vi "Main.vi"() -> (0 "error out":errorcluster)   [LabVIEW 2019]
uses:
  <instrlib>/niDMM/nidmm.llb/niDMM Function.ctl
  <instrlib>/niSwitch/niSwitch.llb/niSwitch Topologies.ctl
  Utility/Result.ctl
  Utility/ErrorOutData.ctl
  <instrlib>/niDCPower/nidcpower.llb/niDCPower Send Software Edge Trigger - Signal.ctl
  <instrlib>/niDMM/nidmm.llb/niDMM Trigger.ctl
  <instrlib>/niDMM/nidmm.llb/niDMM Slope.ctl
  <instrlib>/niDMM/nidmm.llb/niDMM Sample Trigger.ctl
  <instrlib>/niDMM/nidmm.llb/niDMM Control Actions.ctl
  <instrlib>/niDCPower/nidcpower.llb/niDCPower Export Signal - Signal.ctl
  <instrlib>/niDMM/nidmm.llb/niDMM Configure Measurement Absolute.vi
  <instrlib>/niDCPower/nidcpower.llb/niDCPower Configure Software Edge Start Trigger.vi
  <instrlib>/niDCPower/nidcpower.llb/niDCPower Configure Software Edge Sequence Advance Trigger.vi
  <instrlib>/niSwitch/niSwitch.llb/niSwitch Connect Channels (Single).vi
  <instrlib>/niSwitch/niSwitch.llb/niSwitch Disconnect Channels (Single).vi
panel:
  in  "SMU Source Mode":i32(ring)=1021 items=["Single Point"=1020, "Sequence"=1021]
  in  "SMU Output Function":i32(ring)=1007 items=["DC Voltage"=1006, "DC Current"=1007, "Pulse Voltage"=1049, "Pulse Current"=1050]
  in  "SMU Sequence Name":string="MySequence"
  out "Channel Connected":string="ch63"
  in  "Default Results":T1[](array[typedef])
  out "All Results":T1[](array[typedef])=[{"Positive Voltage"=0.05015811388300842, "Positive Current"=0.0, "Negative Voltage"=0.05012649110640674, "Negative Current"=0.0, "Impedance"=inf, "ErrorOutData"={"Error Code"=-2, "Error Message"="\rDMM HI SENSE or LO SENSE lead disconnected\n- DMM measures NaN, or \n- DMM overrange warning, or\n- DMM voltage > DMM Voltage Fault Upper Limit "}}, {"Positive Voltage"=0.05018973665961011, "Positive Current"=0.0, "Negative Voltage"=0.05015811388300842, "Negative Current"=0.0, "Impedance"=inf, "ErrorOutData"={"Error Code"=-2, "Error Message"="\rDMM HI SENSE or LO SENSE lead disconnected\n- DMM measures NaN, or \n- DMM overrange warning, or\n- DMM voltage > DMM Voltage Fault Upper Limit "}}, {"Positive Voltage"=0.05009486832980505, "Positive Current"=0.0, "Negative Voltage"=0.05025298221281347, "Negative Current"=0.0, "Impedance"=-inf, "ErrorOutData"={"Error Code"=-2, "Error Message"="\rDMM HI SENSE or LO SENSE lead disconnected\n- DMM measures NaN, or \n- DMM overrange warning, or\n- DMM voltage > DMM Voltage Fault Upper Limit "}}, {"Positive Voltage"=0.05028460498941516, "Positive Current"=0.0, "Negative Voltage"=0.05, "Negative Current"=0.0, "Impedance"=inf, "ErrorOutData"={"Error Code"=-2, "Error Message"="\rDMM HI SENSE or LO SENSE lead disconnected\n- DMM measures NaN, or \n- DMM overrange warning, or\n- DMM voltage > DMM Voltage Fault Upper Limit "}}, {"Positive Voltage"=0.05025298221281347, "Positive Current"=0.0, "Negative Voltage"=0.05012649110640674, "Negative Current"=0.0, "Impedance"=inf, "ErrorOutData"={"Error Code"=-2, "Error Message"="\rDMM HI SENSE or LO SENSE lead disconnected\n- DMM measures NaN, or \n- DMM overrange warning, or\n- DMM voltage > DMM Voltage Fault Upper Limit "}}, {"Positive Voltage"=0.05015811388300842, "Positive Current"=0.0, "Negative Voltage"=0.05028460498941516, "Negative Current"=0.0, "Impedance"=-inf, "ErrorOutData"={"Error Code"=-2, "Error Message"="\rDMM HI SENSE or LO SENSE lead disconnected\n- DMM measures NaN, or \n- DMM overrange warning, or\n- DMM voltage > DMM Voltage Fault Upper Limit "}}, {"Positive Voltage"=0.05006324555320337, "Positive Current"=0.0, "Negative Voltage"=0.05015811388300842, "Negative Current"=0.0, "Impedance"=-inf, "ErrorOutData"={"Error Code"=-2, "Error Message"="\rDMM HI SENSE or LO SENSE lead disconnected\n- DMM measures NaN, or \n- DMM overrange warning, or\n- DMM voltage > DMM Voltage Fault Upper Limit "}}, {"Positive Voltage"=0.05006324555320337, "Positive Current"=0.0, "Negative Voltage"=0.05006324555320337, "Negative Current"=0.0, "Impedance"=nan, "ErrorOutData"={"Error Code"=-2, "Error Message"="\rDMM HI SENSE or LO SENSE lead disconnected\n- DMM measures NaN, or \n- DMM overrange warning, or\n- DMM voltage > DMM Voltage Fault Upper Limit "}}, {"Positive Voltage"=0.05018973665961011, "Positive Current"=0.0, "Negative Voltage"=0.05022135943621179, "Negative Current"=0.0, "Impedance"=-inf, "ErrorOutData"={"Error Code"=-2, "Error Message"="\rDMM HI SENSE or LO SENSE lead disconnected\n- DMM measures NaN, or \n- DMM overrange warning, or\n- DMM voltage > DMM Voltage Fault Upper Limit "}}, {"Positive Voltage"=0.05006324555320337, "Positive Current"=0.0, "Negative Voltage"=0.05025298221281347, "Negative Current"=0.0, "Impedance"=-inf, "ErrorOutData"={"Error Code"=-2, "Error Message"="\rDMM HI SENSE or LO SENSE lead disconnected\n- DMM measures NaN, or \n- DMM overrange warning, or\n- DMM voltage > DMM Voltage Fault Upper Limit "}}, {"Positive Voltage"=0.05018973665961011, "Positive Current"=0.0, "Negative Voltage"=0.05006324555320337, "Negative Current"=0.0, "Impedance"=inf, "ErrorOutData"={"Error Code"=-2, "Error Message"="\rDMM HI SENSE or LO SENSE lead disconnected\n- DMM measures NaN, or \n- DMM overrange warning, or\n- DMM voltage > DMM Voltage Fault Upper Limit "}}, {"Positive Voltage"=0.050031622776601684, "Positive Current"=0.0, "Negative Voltage"=0.05, "Negative Current"=0.0, "Impedance"=inf, "ErrorOutData"={"Error Code"=-2, "Error Message"="\rDMM HI SENSE or LO SENSE lead disconnected\n- DMM measures NaN, or \n- DMM overrange warning, or\n- DMM voltage > DMM Voltage Fault Upper Limit "}}, {"Positive Voltage"=0.05022135943621179, "Positive Current"=0.0, "Negative Voltage"=0.05015811388300842, "Negative Current"=0.0, "Impedance"=inf, "ErrorOutData"={"Error Code"=-2, "Error Message"="\rDMM HI SENSE or LO SENSE lead disconnected\n- DMM measures NaN, or \n- DMM overrange warning, or\n- DMM voltage > DMM Voltage Fault Upper Limit "}}, {"Positive Voltage"=0.05009486832980505, "Positive Current"=0.0, "Negative Voltage"=0.05009486832980505, "Negative Current"=0.0, "Impedance"=nan, "ErrorOutData"={"Error Code"=-2, "Error Message"="\rDMM HI SENSE or LO SENSE lead disconnected\n- DMM measures NaN, or \n- DMM overrange warning, or\n- DMM voltage > DMM Voltage Fault Upper Limit "}}, {"Positive Voltage"=0.05022135943621179, "Positive Current"=0.0, "Negative Voltage"=0.05025298221281347, "Negative Current"=0.0, "Impedance"=-inf, "ErrorOutData"={"Error Code"=-2, "Error Message"="\rDMM HI SENSE or LO SENSE lead disconnected\n- DMM measures NaN, or \n- DMM overrange warning, or\n- DMM voltage > DMM Voltage Fault Upper Limit "}}, {"Positive Voltage"=0.05028460498941516, "Positive Current"=0.0, "Negative Voltage"=0.05009486832980505, "Negative Current"=0.0, "Impedance"=inf, "ErrorOutData"={"Error Code"=-2, "Error Message"="\rDMM HI SENSE or LO SENSE lead disconnected\n- DMM measures NaN, or \n- DMM overrange warning, or\n- DMM voltage > DMM Voltage Fault Upper Limit "}}, {"Positive Voltage"=0.050031622776601684, "Positive Current"=0.0, "Negative Voltage"=0.05006324555320337, "Negative Current"=0.0, "Impedance"=-inf, "ErrorOutData"={"Error Code"=-2, "Error Message"="\rDMM HI SENSE or LO SENSE lead disconnected\n- DMM measures NaN, or \n- DMM overrange warning, or\n- DMM voltage > DMM Voltage Fault Upper Limit "}}, {"Positive Voltage"=0.05025298221281347, "Positive Current"=0.0, "Negative Voltage"=0.05025298221281347, "Negative Current"=0.0, "Impedance"=nan, "ErrorOutData"={"Error Code"=-2, "Error Message"="\rDMM HI SENSE or LO SENSE lead disconnected\n- DMM measures NaN, or \n- DMM overrange warning, or\n- DMM voltage > DMM Voltage Fault Upper Limit "}}, {"Positive Voltage"=0.05028460498941516, "Positive Current"=0.0, "Negative Voltage"=0.05015811388300842, "Negative Current"=0.0, "Impedance"=inf, "ErrorOutData"={"Error Code"=-2, "Error Message"="\rDMM HI SENSE or LO SENSE lead disconnected\n- DMM measures NaN, or \n- DMM overrange warning, or\n- DMM voltage > DMM Voltage Fault Upper Limit "}}, {"Positive Voltage"=0.05018973665961011, "Positive Current"=0.0, "Negative Voltage"=0.050031622776601684, "Negative Current"=0.0, "Impedance"=inf, "ErrorOutData"={"Error Code"=-2, "Error Message"="\rDMM HI SENSE or LO SENSE lead disconnected\n- DMM measures NaN, or \n- DMM overrange warning, or\n- DMM voltage > DMM Voltage Fault Upper Limit "}}, {"Positive Voltage"=0.05015811388300842, "Positive Current"=0.0, "Negative Voltage"=0.05, "Negative Current"=0.0, "Impedance"=inf, "ErrorOutData"={"Error Code"=-2, "Error Message"="\rDMM HI SENSE or LO SENSE lead disconnected\n- DMM measures NaN, or \n- DMM overrange warning, or\n- DMM voltage > DMM Voltage Fault Upper Limit "}}, {"Positive Voltage"=0.05018973665961011, "Positive Current"=0.0, "Negative Voltage"=0.05015811388300842, "Negative Current"=0.0, "Impedance"=inf, "ErrorOutData"={"Error Code"=-2, "Error Message"="\rDMM HI SENSE or LO SENSE lead disconnected\n- DMM measures NaN, or \n- DMM overrange warning, or\n- DMM voltage > DMM Voltage Fault Upper Limit "}}, {"Positive Voltage"=0.05018973665961011, "Positive Current"=0.0, "Negative Voltage"=0.05028460498941516, "Negative Current"=0.0, "Impedance"=-inf, "ErrorOutData"={"Error Code"=-2, "Error Message"="\rDMM HI SENSE or LO SENSE lead disconnected\n- DMM measures NaN, or \n- DMM overrange warning, or\n- DMM voltage > DMM Voltage Fault Upper Limit "}}, {"Positive Voltage"=0.05018973665961011, "Positive Current"=0.0, "Negative Voltage"=0.05028460498941516, "Negative Current"=0.0, "Impedance"=-inf, "ErrorOutData"={"Error Code"=-2, "Error Message"="\rDMM HI SENSE or LO SENSE lead disconnected\n- DMM measures NaN, or \n- DMM overrange warning, or\n- DMM voltage > DMM Voltage Fault Upper Limit "}}, {"Positive Voltage"=0.05028460498941516, "Positive Current"=0.0, "Negative Voltage"=0.05015811388300842, "Negative Current"=0.0, "Impedance"=inf, "ErrorOutData"={"Error Code"=-2, "Error Message"="\rDMM HI SENSE or LO SENSE lead disconnected\n- DMM measures NaN, or \n- DMM overrange warning, or\n- DMM voltage > DMM Voltage Fault Upper Limit "}}, {"Positive Voltage"=0.05, "Positive Current"=0.0, "Negative Voltage"=0.05022135943621179, "Negative Current"=0.0, "Impedance"=-inf, "ErrorOutData"={"Error Code"=-2, "Error Message"="\rDMM HI SENSE or LO SENSE lead disconnected\n- DMM measures NaN, or \n- DMM overrange warning, or\n- DMM voltage > DMM Voltage Fault Upper Limit "}}, {"Positive Voltage"=0.05, "Positive Current"=0.0, "Negative Voltage"=0.05018973665961011, "Negative Current"=0.0, "Impedance"=-inf, "ErrorOutData"={"Error Code"=-2, "Error Message"="\rDMM HI SENSE or LO SENSE lead disconnected\n- DMM measures NaN, or \n- DMM overrange warning, or\n- DMM voltage > DMM Voltage Fault Upper Limit "}}, {"Positive Voltage"=0.05022135943621179, "Positive Current"=0.0, "Negative Voltage"=0.05028460498941516, "Negative Current"=0.0, "Impedance"=-inf, "ErrorOutData"={"Error Code"=-2, "Error Message"="\rDMM HI SENSE or LO SENSE lead disconnected\n- DMM measures NaN, or \n- DMM overrange warning, or\n- DMM voltage > DMM Voltage Fault Upper Limit "}}, {"Positive Voltage"=0.05009486832980505, "Positive Current"=0.0, "Negative Voltage"=0.05, "Negative Current"=0.0, "Impedance"=inf, "ErrorOutData"={"Error Code"=-2, "Error Message"="\rDMM HI SENSE or LO SENSE lead disconnected\n- DMM measures NaN, or \n- DMM overrange warning, or\n- DMM voltage > DMM Voltage Fault Upper Limit "}}, {"Positive Voltage"=0.05012649110640674, "Positive Current"=0.0, "Negative Voltage"=0.05006324555320337, "Negative Current"=0.0, "Impedance"=inf, "ErrorOutData"={"Error Code"=-2, "Error Message"="\rDMM HI SENSE or LO SENSE lead disconnected\n- DMM measures NaN, or \n- DMM overrange warning, or\n- DMM voltage > DMM Voltage Fault Upper Limit "}}, {"Positive Voltage"=0.05, "Positive Current"=0.0, "Negative Voltage"=0.05, "Negative Current"=0.0, "Impedance"=nan, "ErrorOutData"={"Error Code"=-2, "Error Message"="\rDMM HI SENSE or LO SENSE lead disconnected\n- DMM measures NaN, or \n- DMM overrange warning, or\n- DMM voltage > DMM Voltage Fault Upper Limit "}}, {"Positive Voltage"=0.05, "Positive Current"=0.0, "Negative Voltage"=0.05012649110640674, "Negative Current"=0.0, "Impedance"=-inf, "ErrorOutData"={"Error Code"=-2, "Error Message"="\rDMM HI SENSE or LO SENSE lead disconnected\n- DMM measures NaN, or \n- DMM overrange warning, or\n- DMM voltage > DMM Voltage Fault Upper Limit "}}, {"Positive Voltage"=0.05015811388300842, "Positive Current"=0.0, "Negative Voltage"=0.05018973665961011, "Negative Current"=0.0, "Impedance"=-inf, "ErrorOutData"={"Error Code"=-2, "Error Message"="\rDMM HI SENSE or LO SENSE lead disconnected\n- DMM measures NaN, or \n- DMM overrange warning, or\n- DMM voltage > DMM Voltage Fault Upper Limit "}}, {"Positive Voltage"=0.05015811388300842, "Positive Current"=0.0, "Negative Voltage"=0.05018973665961011, "Negative Current"=0.0, "Impedance"=-inf, "ErrorOutData"={"Error Code"=-2, "Error Message"="\rDMM HI SENSE or LO SENSE lead disconnected\n- DMM measures NaN, or \n- DMM overrange warning, or\n- DMM voltage > DMM Voltage Fault Upper Limit "}}, {"Positive Voltage"=0.05022135943621179, "Positive Current"=0.0, "Negative Voltage"=0.05018973665961011, "Negative Current"=0.0, "Impedance"=inf, "ErrorOutData"={"Error Code"=-2, "Error Message"="\rDMM HI SENSE or LO SENSE lead disconnected\n- DMM measures NaN, or \n- DMM overrange warning, or\n- DMM voltage > DMM Voltage Fault Upper Limit "}}, {"Positive Voltage"=0.05, "Positive Current"=0.0, "Negative Voltage"=0.05018973665961011, "Negative Current"=0.0, "Impedance"=-inf, "ErrorOutData"={"Error Code"=-2, "Error Message"="\rDMM HI SENSE or LO SENSE lead disconnected\n- DMM measures NaN, or \n- DMM overrange warning, or\n- DMM voltage > DMM Voltage Fault Upper Limit "}}, {"Positive Voltage"=0.05028460498941516, "Positive Current"=0.0, "Negative Voltage"=0.05015811388300842, "Negative Current"=0.0, "Impedance"=inf, "ErrorOutData"={"Error Code"=-2, "Error Message"="\rDMM HI SENSE or LO SENSE lead disconnected\n- DMM measures NaN, or \n- DMM overrange warning, or\n- DMM voltage > DMM Voltage Fault Upper Limit "}}, {"Positive Voltage"=0.05009486832980505, "Positive Current"=0.0, "Negative Voltage"=0.05015811388300842, "Negative Current"=0.0, "Impedance"=-inf, "ErrorOutData"={"Error Code"=-2, "Error Message"="\rDMM HI SENSE or LO SENSE lead disconnected\n- DMM measures NaN, or \n- DMM overrange warning, or\n- DMM voltage > DMM Voltage Fault Upper Limit "}}, {"Positive Voltage"=0.05006324555320337, "Positive Current"=0.0, "Negative Voltage"=0.05, "Negative Current"=0.0, "Impedance"=inf, "ErrorOutData"={"Error Code"=-2, "Error Message"="\rDMM HI SENSE or LO SENSE lead disconnected\n- DMM measures NaN, or \n- DMM overrange warning, or\n- DMM voltage > DMM Voltage Fault Upper Limit "}}, {"Positive Voltage"=0.05018973665961011, "Positive Current"=0.0, "Negative Voltage"=0.05018973665961011, "Negative Current"=0.0, "Impedance"=nan, "ErrorOutData"={"Error Code"=-2, "Error Message"="\rDMM HI SENSE or LO SENSE lead disconnected\n- DMM measures NaN, or \n- DMM overrange warning, or\n- DMM voltage > DMM Voltage Fault Upper Limit "}}, {"Positive Voltage"=0.05012649110640674, "Positive Current"=0.0, "Negative Voltage"=0.050031622776601684, "Negative Current"=0.0, "Impedance"=inf, "ErrorOutData"={"Error Code"=-2, "Error Message"="\rDMM HI SENSE or LO SENSE lead disconnected\n- DMM measures NaN, or \n- DMM overrange warning, or\n- DMM voltage > DMM Voltage Fault Upper Limit "}}, {"Positive Voltage"=0.05012649110640674, "Positive Current"=0.0, "Negative Voltage"=0.05, "Negative Current"=0.0, "Impedance"=inf, "ErrorOutData"={"Error Code"=-2, "Error Message"="\rDMM HI SENSE or LO SENSE lead disconnected\n- DMM measures NaN, or \n- DMM overrange warning, or\n- DMM voltage > DMM Voltage Fault Upper Limit "}}, {"Positive Voltage"=0.050031622776601684, "Positive Current"=0.0, "Negative Voltage"=0.05015811388300842, "Negative Current"=0.0, "Impedance"=-inf, "ErrorOutData"={"Error Code"=-2, "Error Message"="\rDMM HI SENSE or LO SENSE lead disconnected\n- DMM measures NaN, or \n- DMM overrange warning, or\n- DMM voltage > DMM Voltage Fault Upper Limit "}}, {"Positive Voltage"=0.05012649110640674, "Positive Current"=0.0, "Negative Voltage"=0.05025298221281347, "Negative Current"=0.0, "Impedance"=-inf, "ErrorOutData"={"Error Code"=-2, "Error Message"="\rDMM HI SENSE or LO SENSE lead disconnected\n- DMM measures NaN, or \n- DMM overrange warning, or\n- DMM voltage > DMM Voltage Fault Upper Limit "}}, {"Positive Voltage"=0.05009486832980505, "Positive Current"=0.0, "Negative Voltage"=0.05028460498941516, "Negative Current"=0.0, "Impedance"=-inf, "ErrorOutData"={"Error Code"=-2, "Error Message"="\rDMM HI SENSE or LO SENSE lead disconnected\n- DMM measures NaN, or \n- DMM overrange warning, or\n- DMM voltage > DMM Voltage Fault Upper Limit "}}, {"Positive Voltage"=0.050031622776601684, "Positive Current"=0.0, "Negative Voltage"=0.05015811388300842, "Negative Current"=0.0, "Impedance"=-inf, "ErrorOutData"={"Error Code"=-2, "Error Message"="\rDMM HI SENSE or LO SENSE lead disconnected\n- DMM measures NaN, or \n- DMM overrange warning, or\n- DMM voltage > DMM Voltage Fault Upper Limit "}}, {"Positive Voltage"=0.05012649110640674, "Positive Current"=0.0, "Negative Voltage"=0.05, "Negative Current"=0.0, "Impedance"=inf, "ErrorOutData"={"Error Code"=-2, "Error Message"="\rDMM HI SENSE or LO SENSE lead disconnected\n- DMM measures NaN, or \n- DMM overrange warning, or\n- DMM voltage > DMM Voltage Fault Upper Limit "}}, {"Positive Voltage"=0.05012649110640674, "Positive Current"=0.0, "Negative Voltage"=0.05022135943621179, "Negative Current"=0.0, "Impedance"=-inf, "ErrorOutData"={"Error Code"=-2, "Error Message"="\rDMM HI SENSE or LO SENSE lead disconnected\n- DMM measures NaN, or \n- DMM overrange warning, or\n- DMM voltage > DMM Voltage Fault Upper Limit "}}, {"Positive Voltage"=0.05025298221281347, "Positive Current"=0.0, "Negative Voltage"=0.05015811388300842, "Negative Current"=0.0, "Impedance"=inf, "ErrorOutData"={"Error Code"=-2, "Error Message"="\rDMM HI SENSE or LO SENSE lead disconnected\n- DMM measures NaN, or \n- DMM overrange warning, or\n- DMM voltage > DMM Voltage Fault Upper Limit "}}, {"Positive Voltage"=0.05028460498941516, "Positive Current"=0.0, "Negative Voltage"=0.05006324555320337, "Negative Current"=0.0, "Impedance"=inf, "ErrorOutData"={"Error Code"=-2, "Error Message"="\rDMM HI SENSE or LO SENSE lead disconnected\n- DMM measures NaN, or \n- DMM overrange warning, or\n- DMM voltage > DMM Voltage Fault Upper Limit "}}, {"Positive Voltage"=0.050031622776601684, "Positive Current"=0.0, "Negative Voltage"=0.05025298221281347, "Negative Current"=0.0, "Impedance"=-inf, "ErrorOutData"={"Error Code"=-2, "Error Message"="\rDMM HI SENSE or LO SENSE lead disconnected\n- DMM measures NaN, or \n- DMM overrange warning, or\n- DMM voltage > DMM Voltage Fault Upper Limit "}}, {"Positive Voltage"=0.05015811388300842, "Positive Current"=0.0, "Negative Voltage"=0.05, "Negative Current"=0.0, "Impedance"=inf, "ErrorOutData"={"Error Code"=-2, "Error Message"="\rDMM HI SENSE or LO SENSE lead disconnected\n- DMM measures NaN, or \n- DMM overrange warning, or\n- DMM voltage > DMM Voltage Fault Upper Limit "}}, {"Positive Voltage"=0.05006324555320337, "Positive Current"=0.0, "Negative Voltage"=0.05009486832980505, "Negative Current"=0.0, "Impedance"=-inf, "ErrorOutData"={"Error Code"=-2, "Error Message"="\rDMM HI SENSE or LO SENSE lead disconnected\n- DMM measures NaN, or \n- DMM overrange warning, or\n- DMM voltage > DMM Voltage Fault Upper Limit "}}, {"Positive Voltage"=0.05012649110640674, "Positive Current"=0.0, "Negative Voltage"=0.05022135943621179, "Negative Current"=0.0, "Impedance"=-inf, "ErrorOutData"={"Error Code"=-2, "Error Message"="\rDMM HI SENSE or LO SENSE lead disconnected\n- DMM measures NaN, or \n- DMM overrange warning, or\n- DMM voltage > DMM Voltage Fault Upper Limit "}}, {"Positive Voltage"=0.05006324555320337, "Positive Current"=0.0, "Negative Voltage"=0.05, "Negative Current"=0.0, "Impedance"=inf, "ErrorOutData"={"Error Code"=-2, "Error Message"="\rDMM HI SENSE or LO SENSE lead disconnected\n- DMM measures NaN, or \n- DMM overrange warning, or\n- DMM voltage > DMM Voltage Fault Upper Limit "}}, {"Positive Voltage"=0.05, "Positive Current"=0.0, "Negative Voltage"=0.05, "Negative Current"=0.0, "Impedance"=nan, "ErrorOutData"={"Error Code"=-2, "Error Message"="\rDMM HI SENSE or LO SENSE lead disconnected\n- DMM measures NaN, or \n- DMM overrange warning, or\n- DMM voltage > DMM Voltage Fault Upper Limit "}}, {"Positive Voltage"=0.05028460498941516, "Positive Current"=0.0, "Negative Voltage"=0.05018973665961011, "Negative Current"=0.0, "Impedance"=inf, "ErrorOutData"={"Error Code"=-2, "Error Message"="\rDMM HI SENSE or LO SENSE lead disconnected\n- DMM measures NaN, or \n- DMM overrange warning, or\n- DMM voltage > DMM Voltage Fault Upper Limit "}}, {"Positive Voltage"=0.050031622776601684, "Positive Current"=0.0, "Negative Voltage"=0.05018973665961011, "Negative Current"=0.0, "Impedance"=-inf, "ErrorOutData"={"Error Code"=-2, "Error Message"="\rDMM HI SENSE or LO SENSE lead disconnected\n- DMM measures NaN, or \n- DMM overrange warning, or\n- DMM voltage > DMM Voltage Fault Upper Limit "}}, {"Positive Voltage"=0.05006324555320337, "Positive Current"=0.0, "Negative Voltage"=0.05006324555320337, "Negative Current"=0.0, "Impedance"=nan, "ErrorOutData"={"Error Code"=-2, "Error Message"="\rDMM HI SENSE or LO SENSE lead disconnected\n- DMM measures NaN, or \n- DMM overrange warning, or\n- DMM voltage > DMM Voltage Fault Upper Limit "}}, {"Positive Voltage"=0.05025298221281347, "Positive Current"=0.0, "Negative Voltage"=0.05015811388300842, "Negative Current"=0.0, "Impedance"=inf, "ErrorOutData"={"Error Code"=-2, "Error Message"="\rDMM HI SENSE or LO SENSE lead disconnected\n- DMM measures NaN, or \n- DMM overrange warning, or\n- DMM voltage > DMM Voltage Fault Upper Limit "}}, {"Positive Voltage"=0.05, "Positive Current"=0.0, "Negative Voltage"=0.05022135943621179, "Negative Current"=0.0, "Impedance"=-inf, "ErrorOutData"={"Error Code"=-2, "Error Message"="\rDMM HI SENSE or LO SENSE lead disconnected\n- DMM measures NaN, or \n- DMM overrange warning, or\n- DMM voltage > DMM Voltage Fault Upper Limit "}}, {"Positive Voltage"=0.05018973665961011, "Positive Current"=0.0, "Negative Voltage"=0.05, "Negative Current"=0.0, "Impedance"=inf, "ErrorOutData"={"Error Code"=-2, "Error Message"="\rDMM HI SENSE or LO SENSE lead disconnected\n- DMM measures NaN, or \n- DMM overrange warning, or\n- DMM voltage > DMM Voltage Fault Upper Limit "}}, {"Positive Voltage"=0.05018973665961011, "Positive Current"=0.0, "Negative Voltage"=0.05018973665961011, "Negative Current"=0.0, "Impedance"=nan, "ErrorOutData"={"Error Code"=-2, "Error Message"="\rDMM HI SENSE or LO SENSE lead disconnected\n- DMM measures NaN, or \n- DMM overrange warning, or\n- DMM voltage > DMM Voltage Fault Upper Limit "}}, {"Positive Voltage"=0.05022135943621179, "Positive Current"=0.0, "Negative Voltage"=0.05015811388300842, "Negative Current"=0.0, "Impedance"=inf, "ErrorOutData"={"Error Code"=-2, "Error Message"="\rDMM HI SENSE or LO SENSE lead disconnected\n- DMM measures NaN, or \n- DMM overrange warning, or\n- DMM voltage > DMM Voltage Fault Upper Limit "}}]
  out "Result":T1={"Positive Voltage"=0.05022135943621179, "Positive Current"=0.0, "Negative Voltage"=0.05015811388300842, "Negative Current"=0.0, "Impedance"=inf, "ErrorOutData"={"Error Code"=-2, "Error Message"="\rDMM HI SENSE or LO SENSE lead disconnected\n- DMM measures NaN, or \n- DMM overrange warning, or\n- DMM voltage > DMM Voltage Fault Upper Limit "}}
  out "Switch Channel List":string[](array[string])=["ch0", "ch1", "ch2", "ch3", "ch4", "ch5", "ch6", "ch7", "ch8", "ch9", "ch10", "ch11", "ch12", "ch13", "ch14", "ch15", "ch16", "ch17", "ch18", "ch19", "ch20", "ch21", "ch22", "ch23", "ch24", "ch25", "ch26", "ch27", "ch28", "ch29", "ch30", "ch31", "ch32", "ch33", "ch34", "ch35", "ch36", "ch37", "ch38", "ch39", "ch40", "ch41", "ch42", "ch43", "ch44", "ch45", "ch46", "ch47", "ch48", "ch49", "ch50", "ch51", "ch52", "ch53", "ch54", "ch55", "ch56", "ch57", "ch58", "ch59", "ch60", "ch61", "ch62", "ch63"]
  in  "SMU Sequence Number of Steps":i32=3
  in  "Sense MUX Switch Topology":T3="2530/2-Wire 64x1 Mux" caption="Sense MUX Topology"
  in  "Sense MUX Switch Resource Name":refnum<k15>="2530B"
  in  "Source MUX Switch Topology":T3="2575/2-Wire 98x1 Mux" caption="Source MUX Topology"
  in  "Source MUX Switch Resource Name":refnum<k15>="2575"
  in  "SMU Sequence Loop Count (Number of Welds)":i32=64
  in  "SMU Source Delay (s)":dbl=0.001 format="%#_13g"
  in  "SMU Measurement Aperture Time (s)":dbl=0.04 format="%#_13g"
  in  "SMU Voltage Limit Range (V)":dbl=6.0 format="%#_13g"
  in  "SMU Voltage Limit (V)":dbl=6.0 format="%#_13g"
  in  "SMU Current Level Range (A)":dbl=1.0 format="%#_13g"
  in  "SMU Current Level (A)":dbl=1.0 format="%#_13g"
  in  "SMU Advanced Sequence Properties":i32[](array[ring])=[1150009, 1150058, 1150051] caption="SMU Advanced Sequence - Step Properties" items=["Source -> Output Function"=1150008, "Source -> Output Enabled"=1250006, "Source -> Output Resistance"=1150061, "Source -> Transient Response"=1150062, "Source -> Custom Transient Response -> Voltage Gain Bandwidth"=1150067, "Source -> Custom Transient Response -> Voltage Compensation Frequency"=1150068, "Source -> Custom Transient Response -> Voltage Pole-Zero Ratio"=1150069, "Source -> Custom Transient Response -> Current Gain Bandwidth"=1150070, "Source -> Custom Transient Response -> Current Compensation Frequency"=1150071, "Source -> Custom Transient Response -> Current Pole-Zero Ratio"=1150072, "Source -> DC Voltage -> Voltage Level"=1250001, "Source -> DC Voltage -> Voltage Level Range"=1150005, "Source -> DC Voltage -> Current Limit"=1250005, "Source -> DC Voltage -> Current Limit High"=1150187, "Source -> DC Voltage -> Current Limit Low"=1150188, "Source -> DC Voltage -> Current Limit Range"=1150004, "Source -> DC Current -> Current Level"=1150009, "Source -> DC Current -> Current Level Range"=1150011, "Source -> DC Current -> Voltage Limit"=1150010, "Source -> DC Current -> Voltage Limit High"=1150185, "Source -> DC Current -> Voltage Limit Low"=1150186, "Source -> DC Current -> Voltage Limit Range"=1150012, "Source -> Pulse Voltage -> Pulse Voltage Level"=1150080, "Source -> Pulse Voltage -> Pulse Bias Voltage Level"=1150082, "Source -> Pulse Voltage -> Pulse Voltage Level Range"=1150084, "Source -> Pulse Voltage -> Pulse Current Limit"=1150081, "Source -> Pulse Voltage -> Pulse Current Limit High"=1150193, "Source -> Pulse Voltage -> Pulse Current Limit Low"=1150194, "Source -> Pulse Voltage -> Pulse Bias Current Limit"=1150083, "Source -> Pulse Voltage -> Pulse Bias Current Limit High"=1150195, "Source -> Pulse Voltage -> Pulse Bias Current Limit Low"=1150196, "Source -> Pulse Voltage -> Pulse Current Limit Range"=1150085, "Source -> Pulse Current -> Pulse Current Level"=1150086, "Source -> Pulse Current -> Pulse Bias Current Level"=1150088, "Source -> Pulse Current -> Pulse Current Level Range"=1150090, "Source -> Pulse Current -> Pulse Voltage Limit"=1150087, "Source -> Pulse Current -> Pulse Voltage Limit High"=1150189, "Source -> Pulse Current -> Pulse Voltage Limit Low"=1150190, "Source -> Pulse Current -> Pulse Bias Voltage Limit"=1150089, "Source -> Pulse Current -> Pulse Bias Voltage Limit High"=1150191, "Source -> Pulse Current -> Pulse Bias Voltage Limit Low"=1150192, "Source -> Pulse Current -> Pulse Voltage Limit Range"=1150091, "Source -> Advanced -> Source Delay"=1150051, "Source -> Advanced -> Pulse Bias Delay"=1150092, "Source -> Advanced -> Pulse On Time"=1150093, "Source -> Advanced -> Pulse Off Time"=1150094, "Source -> Advanced -> OVP Enabled"=1250002, "Source -> Advanced -> OVP Limit"=1250003, "Source -> Advanced -> Compliance Limit Symmetry"=1150184, "Source -> Advanced -> Sequence Step Delta Time"=1150198, "Measurement -> Sense"=1150013, "Measurement -> Aperture Time"=1150058, "Measurement -> Measure Record Length"=1150063, "Measurement -> Advanced -> DC Noise Rejection"=1150066, "Measurement -> Autorange"=1150244, "Measurement -> Advanced -> Autorange Behavior"=1150245, "Measurement -> Advanced -> Autorange Aperture Time Mode"=1150246, "Measurement -> Advanced -> Autorange Minimum Aperture Time"=1150247, "Measurement -> Advanced -> Autorange Minimum Aperture Time Units"=1105248]
  in  "DMM Range (V)":dbl=0.1 format="%#_13g"
  in  "DMM Function":T4
  in  "DMM Resource Name":refnum<k15>="DMM"
  in  "SMU Resource Name":refnum<k15>="SMU"
  in  "DMM Settle Time (s)":dbl=0.002 format="%#_13g"
  in  "DMM Aperture Time (s)":dbl=0.033 format="%#_13g"
  in  "Stop":bool
  out "Channel Index":i32=63
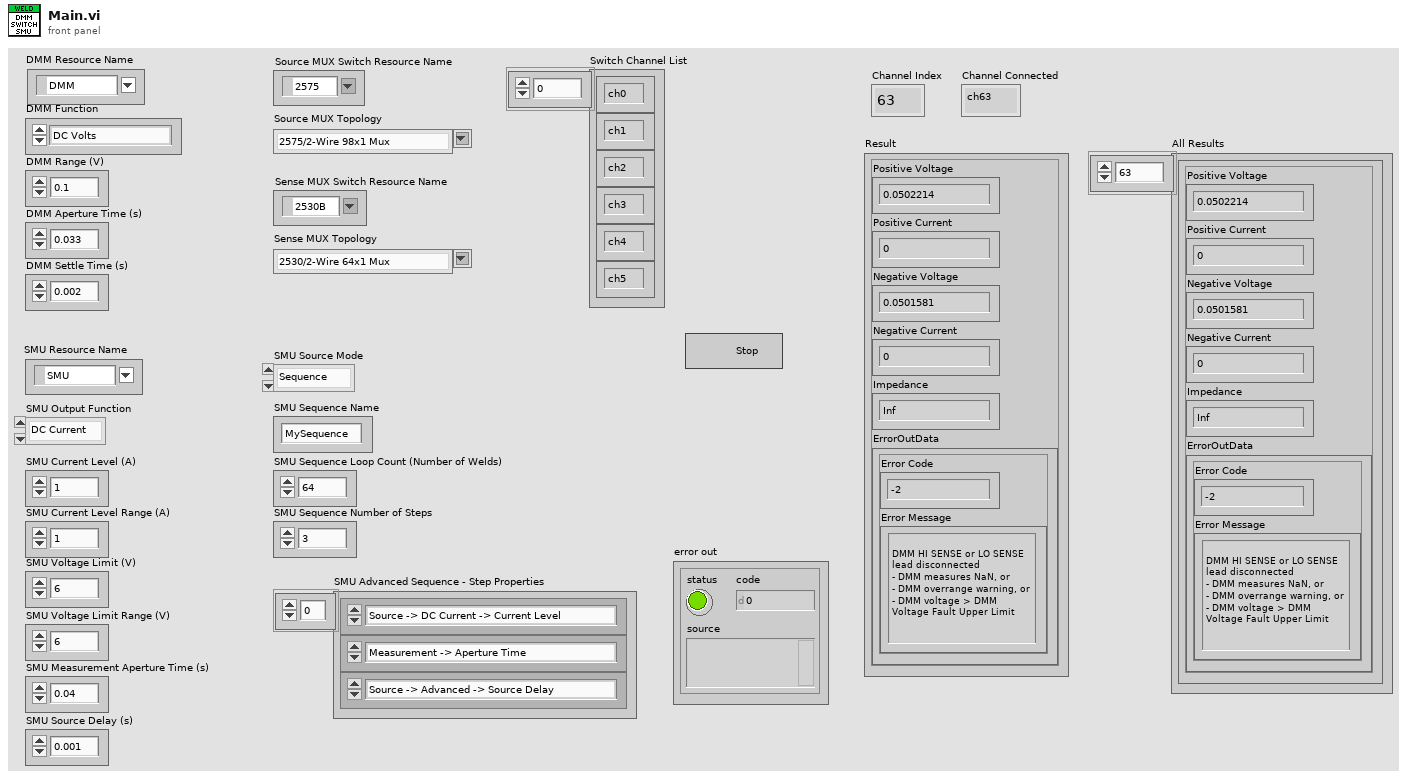
[diagram p1: front panel]
types:
  T1 = typedef "Result.ctl" = cluster{"Positive Voltage":dbl, "Positive Current":dbl, "Negative Voltage":dbl, "Negative Current":dbl, "Impedance":dbl, "ErrorOutData":T2}
  T2 = typedef "ErrorOutData.ctl" = cluster{"Error Code":i32, "Error Message":string}
  T3 = typedef "niSwitch Topologies.ctl" = string
  T4 = typedef "niDMM Function.ctl" = enum16{"DC Volts", "AC Volts", "DC Current", "AC Current", "2-wire Resistance", "4-wire Resistance", "Diode", "Frequency", "Period", "AC Volts DC Coupled", "Capacitance", "Inductance", "Temperature"}
  T5 = typedef "niDCPower Export Signal - Signal.ctl" = i32
  T6 = typedef "niDMM Control Actions.ctl" = i32
  T7 = typedef "niDMM Slope.ctl" = enum16{"Rising Edge", "Falling Edge"}
  T8 = typedef "niDMM Sample Trigger.ctl" = enum16{"Immediate", "External", "TTL 0", "TTL 1", "TTL 2", "TTL 3", "TTL 4", "TTL 5", "TTL 6", "Interval", "Software", "TTL 7", "PXI Star", "LBR Trig 1", "Aux Trig 1"}
  T9 = typedef "niDMM Trigger.ctl" = enum16{"Immediate", "External", "TTL 0", "TTL 1", "TTL 2", "TTL 3", "TTL 4", "TTL 5", "TTL 6", "Software", "TTL 7", "PXI Star", "LBR Trig 1", "Aux Trig 1"}
  T10 = typedef "niDCPower Send Software Edge Trigger - Signal.ctl" = i32
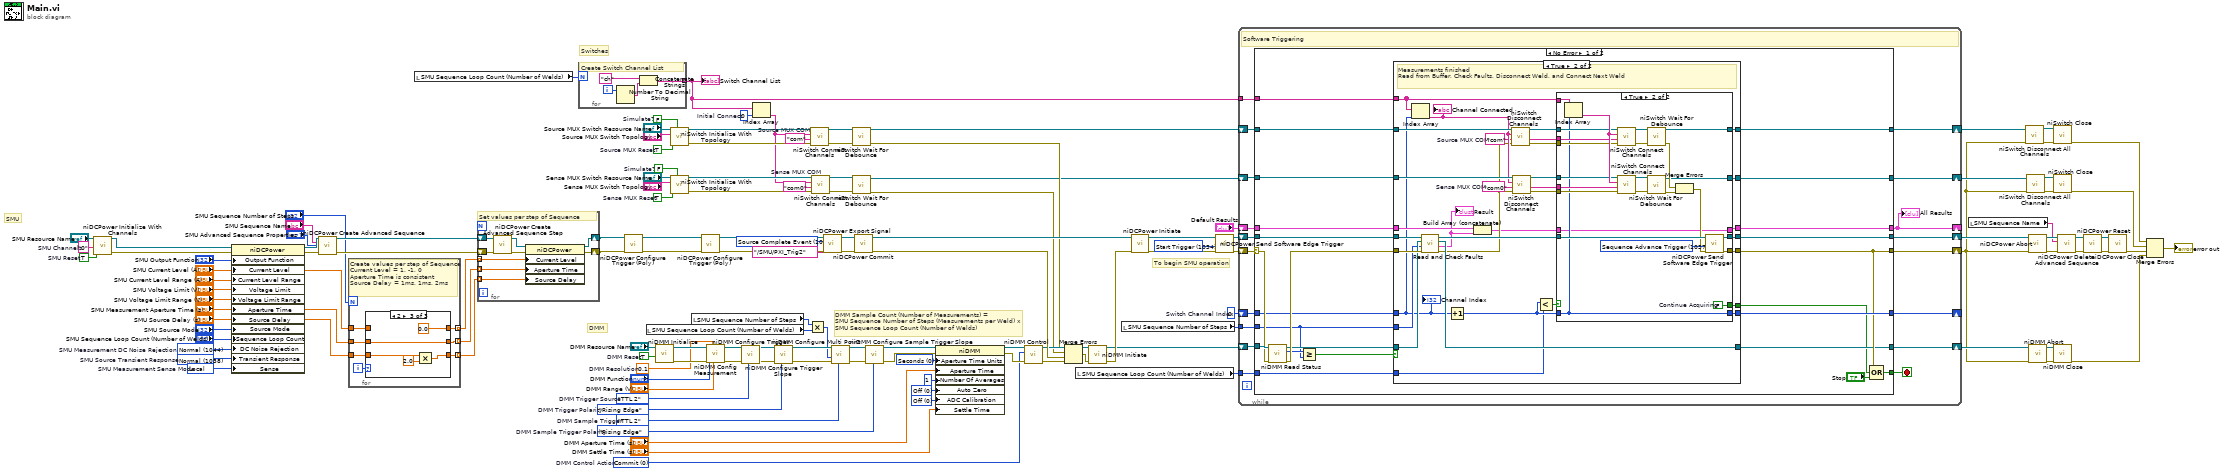
[diagram p0: block diagram]
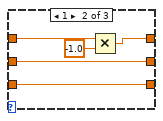
[diagram p3: hidden frame]
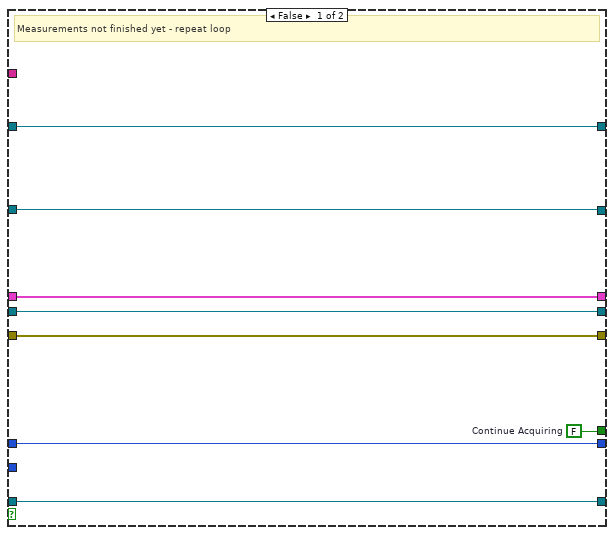
[diagram p4: hidden frame]
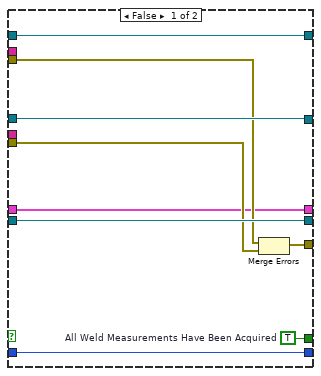
[diagram p5: hidden frame]
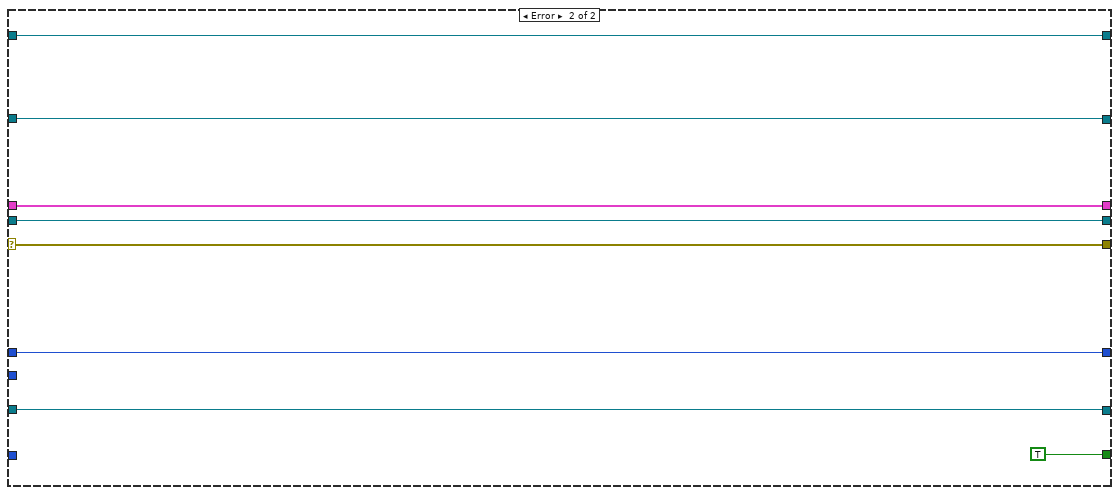
[diagram p6: hidden frame]
diagram:
  w29 = "com0"  # Sense MUX COM
  w30 = 0  # Initial Connect
  w31 = "com"  # Source MUX COM
  w36 = TRUE  # Sense MUX Reset
  w39 = FALSE  # Simulate?
  w40 = TRUE  # Source MUX Reset
  w43 = FALSE  # Simulate?
  w49 = T5 1030 items=["Source Complete Event"=1030, "Measure Complete Event"=1031, "Sequence Iteration Complete Event"=1032, "Sequence Engine Done Event"=1033, "Pulse Complete Event"=1051, "Ready For Pulse Trigger Event"=1052, "Start Trigger"=1034, "Source Trigger"=1035, "Measure Trigger"=1036, "Sequence Advance Trigger"=1037, "Pulse Trigger"=1053] ("signal")
  w65 = 1044 items=["Normal"=1044, "Second-Order"=1043]  # SMU Measurement DC Noise Rejection
  w61 = 1008 items=["Local"=1008, "Remote"=1009]  # SMU Measurement Sense Mode
  w62 = 1038 items=["Slow"=1041, "Normal"=1038, "Fast"=1039, "Custom"=1042]  # SMU Source Transient Response
  w75 = TRUE  # SMU Reset
  w76 = "0"  # SMU Channels
  w79 = 0 items=["Auto"=-1, "Off"=0, "On"=1] ("Configuration:Measurement Options:ADC Calibration")
  w80 = 0 items=["Auto"=-1, "Off"=0, "On"=1, "Once"=2] ("Configuration:Measurement Options:Auto Zero")
  w83 = 0 items=["Seconds", "Power Line Cycles"] ("Configuration:Advanced:Aperture Time Units")
  w84 = T6 0 items=["Commit"]  # DMM Control Action
  w93 = niDMM_Slope."Rising Edge"  # DMM Sample Trigger Polarity
  w97 = niDMM_Sample_Trigger."TTL 2"  # DMM Sample Trigger
  w100 = niDMM_Slope."Rising Edge"  # DMM Trigger Polarity
  w103 = niDMM_Trigger."TTL 2"  # DMM Trigger Source
  w106 = 0.1  # DMM Resolution
  w109 = TRUE  # DMM Reset
  w118 = 0  # Switch Channel Index
  w119 = T10 1034 items=["Start Trigger"=1034, "Source Trigger"=1035, "Measure Trigger"=1036, "Sequence Advance Trigger"=1037, "Pulse Trigger"=1053] ("signal")
  # "DMM Sample Count (Number of Measurements) = \nSMU Sequence Number of Steps (Measurements per Weld) x \nSMU Sequence Loop Count (Number of Welds)"
  # "DMM"
  # "SMU"
  # "Switches"
  # "To begin SMU operation"
  n1 = call <instrlib>:"niDCPower Initialize With Channels.vi"("reset (false)"=w75, "channels"=w76, "resource name"="SMU Resource Name") -> ("error out"=w63:errorcluster, "instrument handle out"=w64:refnum<k15>)  [unwired: 7 in]
  n2 = property class="niDCPower"(reference=w64, error in=w63, "Output Function"="SMU Output Function", "Current Level"="SMU Current Level (A)", "Current Level Range"="SMU Current Level Range (A)", "Voltage Limit"="SMU Voltage Limit (V)", "Voltage Limit Range"="SMU Voltage Limit Range (V)", "Aperture Time"="SMU Measurement Aperture Time (s)", "Source Delay"="SMU Source Delay (s)", "Source Mode"="SMU Source Mode", "Sequence Loop Count"="SMU Sequence Loop Count (Number of Welds)", "DC Noise Rejection"=w65, "Transient Response"=w62, "Sense"=w61) -> (reference out=w72:refnum<k15>, error out=w73:errorcluster)
  n3 = call <instrlib>:"niDCPower Create Advanced Sequence.vi"("instrument handle"=w72, "sequence name"="SMU Sequence Name", "advanced sequence properties"="SMU Advanced Sequence Properties", "error in (no error)"=w73) -> ("instrument handle out"=w60:refnum<k15>, "error out"=w59:errorcluster)  [unwired: 10 in]
  n4 = for {
    N: "SMU Sequence Number of Steps" -> [_]
    tunnel: "SMU Current Level (A)" -> [w141]
    tunnel: [w140] -> w56 mode=indexing
    tunnel: "SMU Measurement Aperture Time (s)" -> [w139]
    tunnel: [w138] -> w44 mode=indexing
    tunnel: "SMU Source Delay (s)" -> [w137]
    tunnel: [w136] -> w53 mode=indexing
    i -> [w142]
    # "Create values per step of Sequence\nCurrent Level = 1, -1, 0\nAperture Time is consistent\nSource Delay = 1ms, 1ms, 2ms"
    n5 = case shown="2" w142 {
      tunnel: w141 -> [w145 w149 _]
      tunnel: [w145 w150 0.0 ("current")] -> w140
      tunnel: w139 -> [w144 w147 w154]
      tunnel: [w144 w147 w154] -> w138
      tunnel: w137 -> [w143 w146 w152]
      tunnel: [w143 w146 w151] -> w136
      frame 0, Default {
      }
      frame 1 {
        n6 = Multiply(x=w149, y=-1.0) -> (x*y=w150:dbl)
      }
      frame 2 {
        n7 = Multiply(x=w152, y=2.0) -> (x*y=w151:dbl)
      }
    }
  }
  n8 = local read "SMU Sequence Loop Count (Number of Welds)"() -> (w34:i32)
  n9 = for {
    shift-right: [w161] -> w51
    shift-left: w59 -> [w164]
    shift-right: [w160] -> w52
    shift-left: w60 -> [w159]
    tunnel: w53 -> [w158] mode=indexing
    tunnel: w56 -> [w156] mode=indexing
    tunnel: w44 -> [w157] mode=indexing
    # "Set values per step of Sequence"
    n10 = call <instrlib>:"niDCPower Create Advanced Sequence Step.vi"("error in (no error)"=w164, "instrument handle"=w159) -> ("error out"=w162:errorcluster, "instrument handle out"=w163:refnum<k15>)  [unwired: 8 in]
    n11 = property class="niDCPower"(reference=w163, error in=w162, "Current Level"=w156, "Aperture Time"=w157, "Source Delay"=w158) -> (reference out=w160:refnum<k15>, error out=w161:errorcluster)
  }
  n12 = for {
    N: w34 -> [_]
    tunnel: [w165] -> w5 mode=indexing
    i -> [w168]
    # "Create Switch Channel List"
    n13 = Number To Decimal String(number=w168) -> (decimal integer string=w166:string)  [unwired: 1 in]
    n14 = Concatenate Strings("ch", w166) -> (w165:string)
  }
  "Switch Channel List" <- w5
  n15 = call-poly <instrlib>:"niDCPower Configure Trigger (Poly).vi"("error in (no error)"=w51, "instrument handle"=w52) -> ("error out"=w134:errorcluster, "instrument handle out"=w135:refnum<k15>)  [unwired: 8 in]
  n16 = local read "SMU Sequence Loop Count (Number of Welds)"() -> (w35:i32)
  n17 = call <instrlib>:"niDMM Initialize.vi"("Reset"=w109, "Instrument Descriptor"="DMM Resource Name") -> ("error out"=w107:errorcluster, "instrument handle out"=w108:refnum<k15>)  [unwired: 8 in]
  n18 = call <instrlib>:"niSwitch Initialize With Topology.vi"("simulate (boolean value)"=w43, "reset device (boolean value)"=w40, "topology name"="Source MUX Switch Topology", "resource name"="Source MUX Switch Resource Name") -> ("error out"=w32:errorcluster, "instrument handle out"=w33:refnum<k15>)  [unwired: 6 in]
  n19 = call <instrlib>:"niSwitch Initialize With Topology.vi"("simulate (boolean value)"=w39, "reset device (boolean value)"=w36, "topology name"="Sense MUX Switch Topology", "resource name"="Sense MUX Switch Resource Name") -> ("error out"=w27:errorcluster, "instrument handle out"=w28:refnum<k15>)  [unwired: 6 in]
  n20 = local read "SMU Sequence Number of Steps"() -> (w2:i32)
  n21 = call-poly <instrlib>:"niDCPower Configure Trigger (Poly).vi"("error in (no error)"=w134, "instrument handle"=w135) -> ("error out"=w47:errorcluster, "instrument handle out"=w50:refnum<k15>)  [unwired: 8 in]
  n22 = call-poly <instrlib>:"niDMM Config Measurement.vi"("Range"="DMM Range (V)", "Resolution"=w106, "error in (no error)"=w107, "Function"="DMM Function", "instrument handle"=w108) -> ("error out"=w102:errorcluster, "instrument handle out"=w101:refnum<k15>)  [unwired: 5 in]
  n23 = call <instrlib>:"niDMM Configure Trigger.vi"("Trigger Source"=w103, "error in (no error)"=w102, "instrument handle"=w101) -> ("error out"=w98:errorcluster, "instrument handle out"=w99:refnum<k15>)  [unwired: 7 in]
  n24 = Index Array(array=w5, index=w30) -> (element=w26:string)
  n25 = call <instrlib>:"niDMM Configure Trigger Slope.vi"("Slope"=w100, "error in (no error)"=w98, "instrument handle"=w99) -> ("error out"=w96:errorcluster, "instrument handle out"=w95:refnum<k15>)  [unwired: 7 in]
  n26 = Multiply(x=w2, y=w35) -> (x*y=w94:i32)
  n27 = call-poly <instrlib>:"niSwitch Connect Channels.vi"("error in (no error)"=w32, "channel 2"=w31, "channel 1"=w26, "instrument handle"=w33) -> ("error out"=w24:errorcluster, "instrument handle out"=w25:refnum<k15>)  [unwired: 6 in]
  n28 = call-poly <instrlib>:"niSwitch Connect Channels.vi"("error in (no error)"=w27, "channel 2"=w29, "channel 1"=w26, "instrument handle"=w28) -> ("error out"=w22:errorcluster, "instrument handle out"=w23:refnum<k15>)  [unwired: 6 in]
  n29 = call <instrlib>:"niDCPower Export Signal.vi"("error in (no error)"=w47, "output terminal"=tag "/SMU/PXI_Trig2", "signal"=w49, "instrument handle"=w50) -> ("error out"=w45:errorcluster, "instrument handle out"=w46:refnum<k15>)  [unwired: 6 in]
  n30 = call <instrlib>:"niDMM Configure Multi Point.vi"("Sample Trigger"=w97, "error in (no error)"=w96, "Sample Count"=w94, "instrument handle"=w95) -> ("error out"=w91:errorcluster, "instrument handle out"=w92:refnum<k15>)  [unwired: 6 in]
  n31 = call <instrlib>:"niSwitch Wait For Debounce.vi"("error in (no error)"=w24, "instrument handle"=w25) -> ("error out"=w20:errorcluster, "instrument handle out"=w16:refnum<k15>)  [unwired: 8 in]
  n32 = call <instrlib>:"niSwitch Wait For Debounce.vi"("error in (no error)"=w22, "instrument handle"=w23) -> ("error out"=w21:errorcluster, "instrument handle out"=w17:refnum<k15>)  [unwired: 8 in]
  n33 = call <instrlib>:"niDCPower Commit.vi"("error in (no error)"=w45, "instrument handle"=w46) -> ("error out"=w125:errorcluster, "instrument handle out"=w123:refnum<k15>)  [unwired: 8 in]
  n34 = call <instrlib>:"niDMM Configure Sample Trigger Slope.vi"("Slope"=w93, "error in (no error)"=w91, "instrument handle"=w92) -> ("error out"=w85:errorcluster, "instrument handle out"=w88:refnum<k15>)  [unwired: 7 in]
  n35 = property class="niDMM"(reference=w88, error in=w85, "Aperture Time Units"=w83, "Aperture Time"="DMM Aperture Time (s)", "Number Of Averages"=1 ("Configuration:Advanced:Number Of Averages"), "Auto Zero"=w80, "ADC Calibration"=w79, "Settle Time"="DMM Settle Time (s)") -> (reference out=w89:refnum<k15>, error out=w90:errorcluster)
  n36 = call <instrlib>:"niDMM Control.vi"("error in (no error)"=w90, "Control Action"=w84, "instrument handle"=w89) -> ("error out"=w86:errorcluster, "instrument handle out"=w87:refnum<k15>)  [unwired: 7 in]
  n37 = Merge Errors(w20, w21, w125, w86) -> (w124:errorcluster)
  n38 = local read "SMU Sequence Loop Count (Number of Welds)"() -> (w1:i32)
  n39 = call <instrlib>:"niDMM Initiate.vi"("error in (no error)"=w124, "instrument handle"=w87) -> ("error out"=w116:errorcluster, "instrument handle out"=w114:refnum<k15>)  [unwired: 8 in]
  n40 = local read "SMU Sequence Number of Steps"() -> (w19:i32)
  n41 = call <instrlib>:"niDCPower Initiate.vi"("error in (no error)"=w116, "instrument handle"=w123) -> ("error out"=w117:errorcluster, "instrument handle out"=w120:refnum<k15>)  [unwired: 8 in]
  n42 = call <instrlib>:"niDCPower Send Software Edge Trigger.vi"("error in (no error)"=w117, "signal"=w119, "instrument handle"=w120) -> ("error out"=w113:errorcluster, "instrument handle out"=w115:refnum<k15>)  [unwired: 7 in]
  n43 = while {
    shift-right: [w186] -> w111
    shift-left: w115 -> [w185]
    shift-right: [w180] -> w9
    shift-left: w113 -> [w178]
    shift-right: [w182] -> w110
    shift-left: w114 -> [w183]
    shift-right: [w184] -> _
    shift-left: w118 -> [w181]
    shift-right: [w175] -> _
    shift-left: "Default Results" -> [w177]
    tunnel: w19 -> [w176]
    tunnel: w5 -> [w172]
    shift-right: [w171] -> w13
    shift-left: w16 -> [w173]
    shift-right: [w170] -> w10
    shift-left: w17 -> [w174]
    tunnel: w1 -> [w169]
    stop <- w179 stop-if-true
    # "Software Triggering"
    n44 = case shown="No Error" w178 {
      selector: w178 -> [w206 w287]
      tunnel: [w199 w286] -> w186
      tunnel: w185 -> [w210 w286]
      tunnel: [w209 w288] -> w184
      tunnel: w183 -> [w208 w289]
      tunnel: [w198 w289] -> w182
      tunnel: w181 -> [w205 w288]
      tunnel: [w201 w287] -> w180
      tunnel: [w204 TRUE] -> w179
      tunnel: w177 -> [w202 w285]
      tunnel: [w200 w285] -> w175
      tunnel: w176 -> [w194 _]
      tunnel: w174 -> [w193 w284]
      tunnel: w173 -> [w192 w283]
      tunnel: w172 -> [w191 _]
      tunnel: [w190 w283] -> w171
      tunnel: [w189 w284] -> w170
      tunnel: w169 -> [w187 _]
      frame No Error {
        n45 = call <instrlib>:"niDMM Read Status.vi"("error in (no error)"=w206, "instrument handle"=w208) -> ("error out"=w207:errorcluster, "Backlog"=w196:i32, "instrument handle out"=w203:refnum<k15>)  [unwired: 6 in, 1 out]
        n46 = Greater Or Equal?(x=w196, y=w194) -> (x >= y?=w195:bool)
        n47 = case shown="True" w195 {
          tunnel: w207 -> [w217 w246]
          tunnel: [w218 w249] -> w199
          tunnel: [w217 w248] -> w201
          tunnel: w210 -> [w218 w247]
          tunnel: w205 -> [w216 w234]
          tunnel: [w216 w225] -> w209
          tunnel: w203 -> [w215 w244]
          tunnel: [w215 w243] -> w198
          tunnel: w202 -> [w214 w242]
          tunnel: [w214 w223] -> w200
          tunnel: w194 -> [_ w241]
          tunnel: w193 -> [w212 w237]
          tunnel: w192 -> [w213 w239]
          tunnel: w191 -> [_ w235]
          tunnel: [w213 w229] -> w190
          tunnel: [w212 w228] -> w189
          tunnel: [w211 w222] -> w188
          tunnel: w187 -> [_ w219]
          frame False {
            w211 = FALSE  # Continue Acquiring
            # "Measurements not finished yet - repeat loop"
          }
          frame True {
            w226 = "com0"  # Sense MUX COM
            w227 = "com"  # Source MUX COM
            # "Measurements finished\nRead from Buffer, Check Faults, Disconnect Weld, and Connect Next Weld"
            n48 = Index Array(array=w235, index=w234) -> (element=w233:string)
            "Channel Connected" <- w233
            n49 = call "Read and Check Faults.vi"("error in (no error)"=w246, "SMUSequenceNumberOfSteps"=w241, "DMM Ref"=w244, "SMU Ref"=w247) -> ("error out"=w232:errorcluster, "Result"=w240:T1, "DMM Ref Out"=w243:refnum<k15>, "SMU Ref Out"=w245:refnum<k15>)  [unwired: 4 in]
            "Result" <- w240
            n50 = Increment(x=w234) -> (x+1=w220:i32)
            n51 = Build Array (concatenate)(w242, w240) -> (w224:T1[])
            n52 = call-poly <instrlib>:"niSwitch Disconnect Channels.vi"("error in (no error)"=w232, "channel 2"=w227, "channel 1"=w233, "instrument handle"=w239) -> ("error out"=w231:errorcluster, "instrument handle out"=w238:refnum<k15>)  [unwired: 6 in]
            n53 = call-poly <instrlib>:"niSwitch Disconnect Channels.vi"("error in (no error)"=w232, "channel 2"=w226, "channel 1"=w233, "instrument handle"=w237) -> ("error out"=w230:errorcluster, "instrument handle out"=w236:refnum<k15>)  [unwired: 6 in]
            n54 = Less?(x=w220, y=w219) -> (x < y?=w221:bool)
            n55 = case shown="True" w221 {
              tunnel: [w256 w282] -> w249
              tunnel: [w255 w281] -> w248
              tunnel: w245 -> [w256 w279]
              tunnel: w238 -> [w258 w273]
              tunnel: w236 -> [w257 w272]
              tunnel: w220 -> [w251 w261]
              tunnel: w235 -> [_ w271]
              tunnel: w231 -> [w254 w270]
              tunnel: w230 -> [w253 w269]
              tunnel: [w258 w266] -> w229
              tunnel: [w257 w265] -> w228
              tunnel: w227 -> [_ w263]
              tunnel: w226 -> [_ w262]
              tunnel: [w251 w261] -> w225
              tunnel: w224 -> [w252 w260]
              tunnel: [w252 w260] -> w223
              tunnel: [w250 w259] -> w222
              frame False {
                w250 = TRUE  # All Weld Measurements Have Been Acquired
                n56 = Merge Errors(w254, w253) -> (w255:errorcluster)
              }
              frame True {
                w259 = FALSE  # Continue Acquiring
                w280 = T10 1037 items=["Start Trigger"=1034, "Source Trigger"=1035, "Measure Trigger"=1036, "Sequence Advance Trigger"=1037, "Pulse Trigger"=1053] ("signal")
                n57 = Index Array(array=w271, index=w261) -> (element=w278:string)
                n58 = call-poly <instrlib>:"niSwitch Connect Channels.vi"("error in (no error)"=w270, "channel 2"=w263, "channel 1"=w278, "instrument handle"=w273) -> ("error out"=w276:errorcluster, "instrument handle out"=w277:refnum<k15>)  [unwired: 6 in]
                n59 = call-poly <instrlib>:"niSwitch Connect Channels.vi"("error in (no error)"=w269, "channel 2"=w262, "channel 1"=w278, "instrument handle"=w272) -> ("error out"=w274:errorcluster, "instrument handle out"=w275:refnum<k15>)  [unwired: 6 in]
                n60 = call <instrlib>:"niSwitch Wait For Debounce.vi"("error in (no error)"=w276, "instrument handle"=w277) -> ("error out"=w267:errorcluster, "instrument handle out"=w266:refnum<k15>)  [unwired: 8 in]
                n61 = call <instrlib>:"niSwitch Wait For Debounce.vi"("error in (no error)"=w274, "instrument handle"=w275) -> ("error out"=w268:errorcluster, "instrument handle out"=w265:refnum<k15>)  [unwired: 8 in]
                n62 = Merge Errors(w267, w268) -> (w264:errorcluster)
                n63 = call <instrlib>:"niDCPower Send Software Edge Trigger.vi"("error in (no error)"=w264, "signal"=w280, "instrument handle"=w279) -> ("error out"=w281:errorcluster, "instrument handle out"=w282:refnum<k15>)  [unwired: 7 in]
              }
            }
            "Channel Index" <- w234
          }
        }
        n64 = Compound Arithmetic op=OR(w201, w188, "Stop") -> (w204:bool)
      }
      frame Error {
      }
    }
    "All Results" <- w175
  }
  n65 = local read "SMU Sequence Name"() -> (w8:string)
  n66 = call <instrlib>:"niSwitch Disconnect All Channels.vi"("error in (no error)"=w9, "instrument handle"=w13) -> ("error out"=w15:errorcluster, "instrument handle out"=w14:refnum<k15>)  [unwired: 8 in]
  n67 = call <instrlib>:"niSwitch Disconnect All Channels.vi"("error in (no error)"=w9, "instrument handle"=w10) -> ("error out"=w12:errorcluster, "instrument handle out"=w11:refnum<k15>)  [unwired: 8 in]
  n68 = call <instrlib>:"niDCPower Abort.vi"("error in (no error)"=w9, "instrument handle"=w111) -> ("error out"=w132:errorcluster, "instrument handle out"=w133:refnum<k15>)  [unwired: 8 in]
  n69 = call <instrlib>:"niDMM Abort.vi"("error in (no error)"=w9, "instrument handle"=w110) -> ("error out"=w127:errorcluster, "instrument handle out"=w126:refnum<k15>)  [unwired: 8 in]
  n70 = call <instrlib>:"niSwitch Close.vi"("error in (no error)"=w15, "instrument handle"=w14) -> ("error out"=w6:errorcluster)  [unwired: 9 in]
  n71 = call <instrlib>:"niSwitch Close.vi"("error in (no error)"=w12, "instrument handle"=w11) -> ("error out"=w7:errorcluster)  [unwired: 9 in]
  n72 = call <instrlib>:"niDMM Close.vi"("error in (no error)"=w127, "instrument handle"=w126) -> ("error out"=w122:errorcluster)  [unwired: 9 in]
  n73 = call <instrlib>:"niDCPower Delete Advanced Sequence.vi"("error in (no error)"=w132, "sequence name"=w8, "instrument handle"=w133) -> ("error out"=w131:errorcluster, "instrument handle out"=w130:refnum<k15>)  [unwired: 7 in]
  n74 = call <instrlib>:"niDCPower Reset.vi"("error in (no error)"=w131, "instrument handle"=w130) -> ("error out"=w128:errorcluster, "instrument handle out"=w129:refnum<k15>)  [unwired: 2 in, 6 out]
  n75 = call <instrlib>:"niDCPower Close.vi"("error in (no error)"=w128, "instrument handle"=w129) -> ("error out"=w121:errorcluster)  [unwired: 9 in]
  n76 = Merge Errors(w6, w7, w121, w122) -> (→"error out":errorcluster)
